vi "4.feladat.vi"() -> ()   [LabVIEW 2015]
panel:
  out "Az átváltó futási ideje":dbl
  out "Csak a for ciklus futási ideje":dbl
  out "For ciklus + átváltás futási ideje":dbl
  # "A kettõ különbségébõl:"
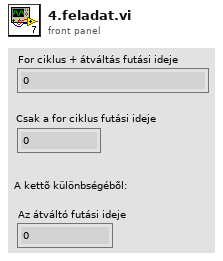
[diagram p1: front panel]
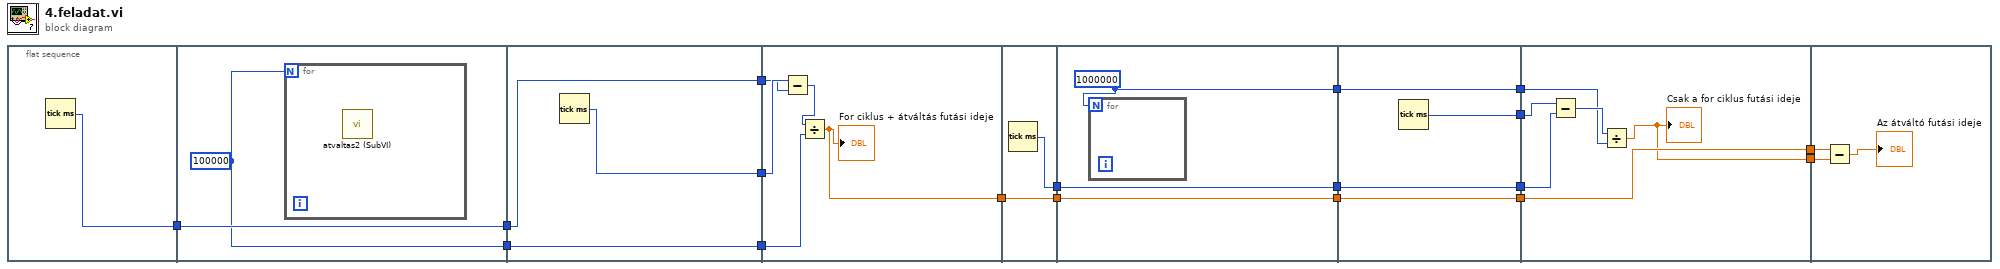
[diagram p0: block diagram]
diagram:
  n1 = flat-sequence {
    tunnel: [w19] -> w17
    tunnel: [w21] -> w18
    tunnel: w17 -> [w21]
    tunnel: [w20] -> w16
    tunnel: w18 -> [w23]
    tunnel: w16 -> [w22]
    tunnel: [w24] -> w15
    tunnel: [w23] -> w14
    tunnel: [w22] -> w13
    tunnel: w15 -> [w27]
    tunnel: w14 -> [w26]
    tunnel: w13 -> [w28]
    tunnel: [w25] -> w2
    tunnel: [w31] -> w10
    tunnel: [w30] -> w3
    tunnel: w2 -> [w30]
    tunnel: [w34] -> w11
    tunnel: w10 -> [w34]
    tunnel: [w33] -> w7
    tunnel: [w32] -> w4
    tunnel: w3 -> [w32]
    tunnel: [w38] -> w12
    tunnel: w11 -> [w38]
    tunnel: [w37] -> w9
    tunnel: [w36] -> w8
    tunnel: w7 -> [w36]
    tunnel: [w35] -> w5
    tunnel: w4 -> [w35]
    tunnel: w12 -> [w41]
    tunnel: w9 -> [w42]
    tunnel: w8 -> [w43]
    tunnel: [w40] -> w6
    tunnel: w5 -> [w40]
    tunnel: [w39] -> w1
    tunnel: w6 -> [w47]
    tunnel: w1 -> [w46]
    frame #0 {
      n2 = Tick Count (ms)() -> (millisecond timer value=w19:u32)
    }
    frame #1 {
      w20 = 100000
      n3 = for {
        N: w20 -> [_]
        n4 = call "atvaltas2 (SubVI).vi"() -> ()  [unwired: 11 in, 1 out]
      }
    }
    frame #2 {
      n5 = Tick Count (ms)() -> (millisecond timer value=w24:u32)
    }
    frame #3 {
      n6 = Subtract(x=w27, y=w26) -> (x-y=w29:u32)
      n7 = Divide(x=w29, y=w28) -> (x/y=w25:dbl)
      "For ciklus + átváltás futási ideje" <- w25
    }
    frame #4 {
      n8 = Tick Count (ms)() -> (millisecond timer value=w31:u32)
    }
    frame #5 {
      w33 = 1000000
      n9 = for {
        N: w33 -> [_]
      }
    }
    frame #6 {
      n10 = Tick Count (ms)() -> (millisecond timer value=w37:u32)
    }
    frame #7 {
      n11 = Subtract(x=w42, y=w41) -> (x-y=w44:u32)
      n12 = Divide(x=w44, y=w43) -> (x/y=w39:dbl)
      "Csak a for ciklus futási ideje" <- w39
    }
    frame #8 {
      n13 = Subtract(x=w47, y=w46) -> (x-y=→"Az átváltó futási ideje":dbl)
    }
  }
